vi "XBOX_Control_Msg.vi"(8 "error in (no error)":errorcluster caption="错误输入（无错误）", 10 "XBOX_Control":T1, 11 "Manual 输入":refnum<class "Manual.lvclass">) -> (0 "error out":errorcluster caption="错误输出", 3 "Process State out":refnum<class "State Actor.lvclass">)   [LabVIEW 2014, in "States.lvlib" / "Manual.lvclass"]
doc: "在Manual模式中，将手柄指令进行计算转化为速度值\n发送给P3AT操作者，P3AT发送给ROS"
uses:
  Manual.lvclass
  <vilib>/NI/Actors/State Actor/State Actor/State Actor.lvclass
  ctl/XBOX_Control.ctl
  <vilib>/MakerHub/Xbox-One-Controller/Private/Type Defs/Indicators/All Buttons Visual.ctl
  <vilib>/MakerHub/Xbox-One-Controller/Private/Type Defs/Indicators/A.ctl
  <vilib>/MakerHub/Xbox-One-Controller/Private/Type Defs/Indicators/B.ctl
  <vilib>/MakerHub/Xbox-One-Controller/Private/Type Defs/Indicators/X.ctl
  <vilib>/MakerHub/Xbox-One-Controller/Private/Type Defs/Indicators/Y.ctl
  <vilib>/MakerHub/Xbox-One-Controller/Private/Type Defs/Indicators/Left Bumper.ctl
  <vilib>/MakerHub/Xbox-One-Controller/Private/Type Defs/Indicators/Right Bumper.ctl
  <vilib>/MakerHub/Xbox-One-Controller/Private/Type Defs/Indicators/View.ctl
  <vilib>/MakerHub/Xbox-One-Controller/Private/Type Defs/Indicators/Menu.ctl
  <vilib>/MakerHub/Xbox-One-Controller/Private/Type Defs/Indicators/Thumbstick.ctl
  <vilib>/MakerHub/Xbox-One-Controller/Private/Type Defs/Indicators/All Axis Data.ctl
  <vilib>/MakerHub/Xbox-One-Controller/Private/Type Defs/Indicators/DPad Enum.ctl
  <vilib>/ActorFramework/Message Enqueuer/Message Enqueuer.lvclass/Message Enqueuer.ctl
  <vilib>/ActorFramework/Message Enqueuer/Enqueue.vi
  <vilib>/ActorFramework/Message Priority Queue/Priority Enqueue.vi
  <vilib>/MakerHub/Xbox-One-Controller/LMH-Xbox-One-Controller.lvlib
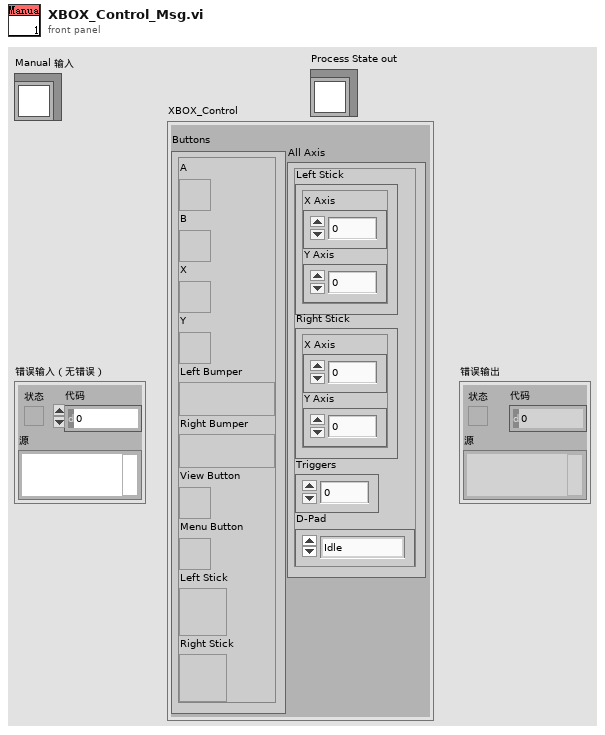
[diagram p1: front panel]
types:
  T1 = typedef "XBOX_Control.ctl" = cluster{"Buttons":T2, "All Axis":T12}
  T2 = typedef "LMH-Xbox-One-Controller.lvlib/All Buttons Visual.ctl" = cluster{"A":T3, "B":T4, "X":T5, "Y":T6, "Left Bumper":T7, "Right Bumper":T8, "View Button":T9, "Menu Button":T10, "Left Stick":T11, "Right Stick":T11}
  T3 = typedef "LMH-Xbox-One-Controller.lvlib/A.ctl" = bool
  T4 = typedef "LMH-Xbox-One-Controller.lvlib/B.ctl" = bool
  T5 = typedef "LMH-Xbox-One-Controller.lvlib/X.ctl" = bool
  T6 = typedef "LMH-Xbox-One-Controller.lvlib/Y.ctl" = bool
  T7 = typedef "LMH-Xbox-One-Controller.lvlib/Left Bumper.ctl" = bool
  T8 = typedef "LMH-Xbox-One-Controller.lvlib/Right Bumper.ctl" = bool
  T9 = typedef "LMH-Xbox-One-Controller.lvlib/View.ctl" = bool
  T10 = typedef "LMH-Xbox-One-Controller.lvlib/Menu.ctl" = bool
  T11 = typedef "LMH-Xbox-One-Controller.lvlib/Thumbstick.ctl" = bool
  T12 = typedef "LMH-Xbox-One-Controller.lvlib/All Axis Data.ctl" = cluster{"Left Stick":cluster{"X Axis":i32, "Y Axis":i32}, "Right Stick":cluster{"X Axis":i32, "Y Axis":i32}, "Triggers":i32, "D-Pad":T13}
  T13 = typedef "LMH-Xbox-One-Controller.lvlib/DPad Enum.ctl" = enum16{"Idle", "Up", "Up / Right", "Right", "Down / Right", "Down", "Down / Left", "Left", "Up / Left"}
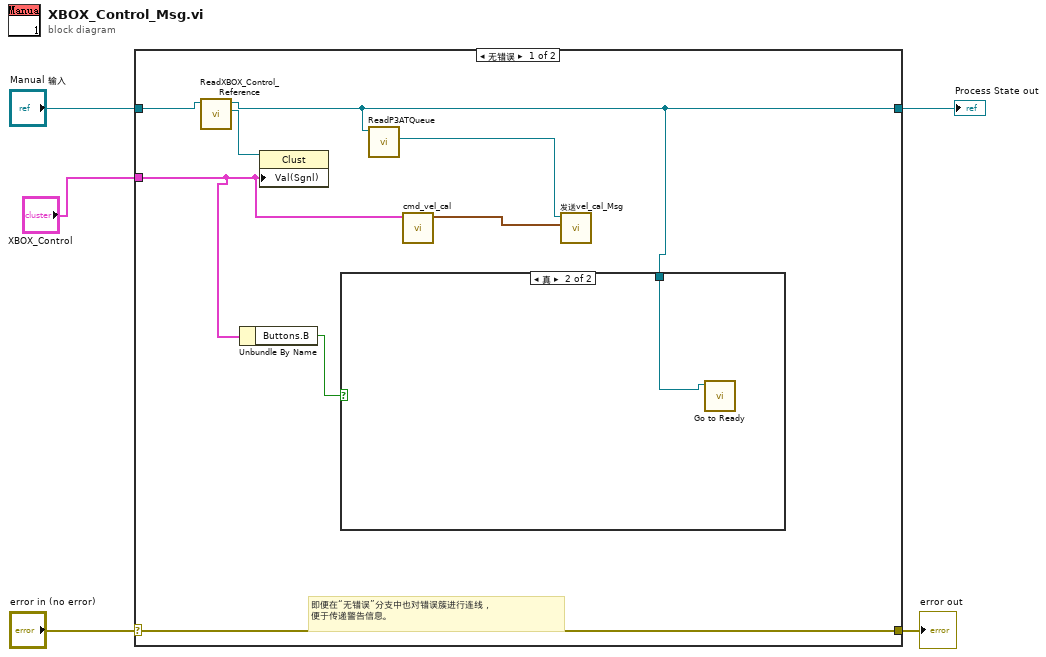
[diagram p0: block diagram]
diagram:
  n1 = case shown="无错误" "error in (no error)" {
    selector: "error in (no error)" -> [w13 w16]
    tunnel: [w13 w16] -> w4
    tunnel: [w6 w15] -> w2
    tunnel: "Manual 输入" -> [w12 w15]
    tunnel: "XBOX_Control" -> [w7 _]
    frame No Error {
      # "即便在“无错误”分支中也对错误簇进行连线，\n便于传递警告信息。"
      n2 = call-dynamic "ReadXBOX_Control_Reference.vi"("CoordinatorState输入"=w12) -> ("XBOX_Control_Reference"=w11:refnum<vi>, "CoordinatorState输出"=w6:refnum<class "Manual.lvclass">)  [unwired: 8 in, 1 out]
      n3 = Unbundle By Name(w7) -> ("Buttons.B"=w8:T4)
      n4 = property class="Clust"(reference=w11, "Val(Sgnl)"=w7) -> ()  [unwired: 1 in, 2 out]
      n5 = case shown="真" w8 {
        tunnel: w6 -> [_ w14]
        frame False {
        }
        frame True {
          n6 = call-dynamic "Go to Ready.vi"("CommonState in"=w14) -> ()  [unwired: 9 in, 2 out]
        }
      }
      n7 = call-dynamic "ReadP3ATQueue.vi"("CoordinatorState输入"=w6) -> ("操作者框架:消息待入队列"=w9:refnum<class "Message Enqueuer.lvclass">)  [unwired: 8 in, 2 out]
      n8 = call "cmd_vel_cal.vi"("XBOX_Control"=w7) -> ("vel_cal"=w10:cluster{"rot_z":dbl, "lin_x":dbl})  [unwired: 8 in]
      n9 = call "发送vel_cal_Msg.vi"("值(信号)"=w10, "消息待入队列"=w9) -> ()  [unwired: 8 in, 2 out]
    }
    frame Error {
    }
  }
  "error out" <- w4
  "Process State out" <- w2
